vi "Read Images from File.vi"() -> ()   [LabVIEW 2023]
doc: "The Read Images from File example shows how to read images from various file types. These include a folder of image formats such as PNG, JPG, BMP, and TIFF, as well as AVI and TDMS. Use the Comparison of Streaming File Formats, Stream to AVI, Stream to Image File, or Stream to TDMS examples to create these image files."
uses:
  <vilib>/vision/Avi.llb/IMAQ AVI2 Refnum.ctl
  SubVIs/TDMS Read Data.ctl
  <vilib>/vision/Image Controls.llb/IMAQ Image.ctl
  SubVIs/TDMS File Initialization (Read).vi
panel:
  in  "Stop":bool
  in  "Image Type":u16(ring) items=["Grayscale (U8)"=0, "Grayscale (I16)"=1, "Grayscale (U16)"=7, "RGB Color (U32)"=4]
  in  "Selected Image Index":u64(slide) scale=0.0..1196.0
  out "Image":T1(plugin-control)
  in  "File Path":path
  # "Overview: Demonstrates how to read images from various file formats: image files (i.e. PNG, BMP, TIFF, etc.), AVI, and TDMS.\nRequirements: Vision Acquisition Software\nInstructions:\n1. Select the File Path to the image file to read. For image files, all images of the same type in the folder will also be read.\n2. Select the Image Type of the images saved in the file for TDMS file types. Other file types don't require this.\n3. Run the VI"
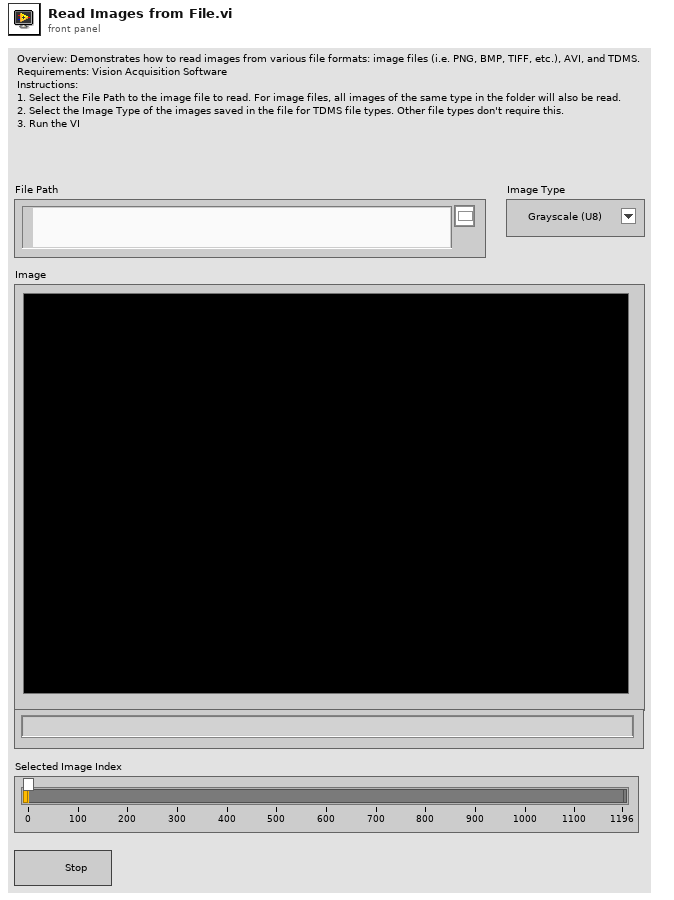
[diagram p1: front panel]
types:
  T1 = typedef "IMAQ Image.ctl" = refnum<image>
  T2 = typedef "IMAQ AVI2 Refnum.ctl" = refnum<k20>
  T3 = typedef "TDMS Read Data.ctl" = cluster{"Image Type":T4, "Width":u32, "Height":u32, "Pixels per Image":u32, "Total Width":u32, "Left Offset":u32, "Image":T1}
  T4 = typedef "Image Type" = u32
  T5 = cluster{"Image File Paths":path[], "AVI Ref":T2, "TDMS Ref":refnum<k34>, "TDMS Settings":T3}
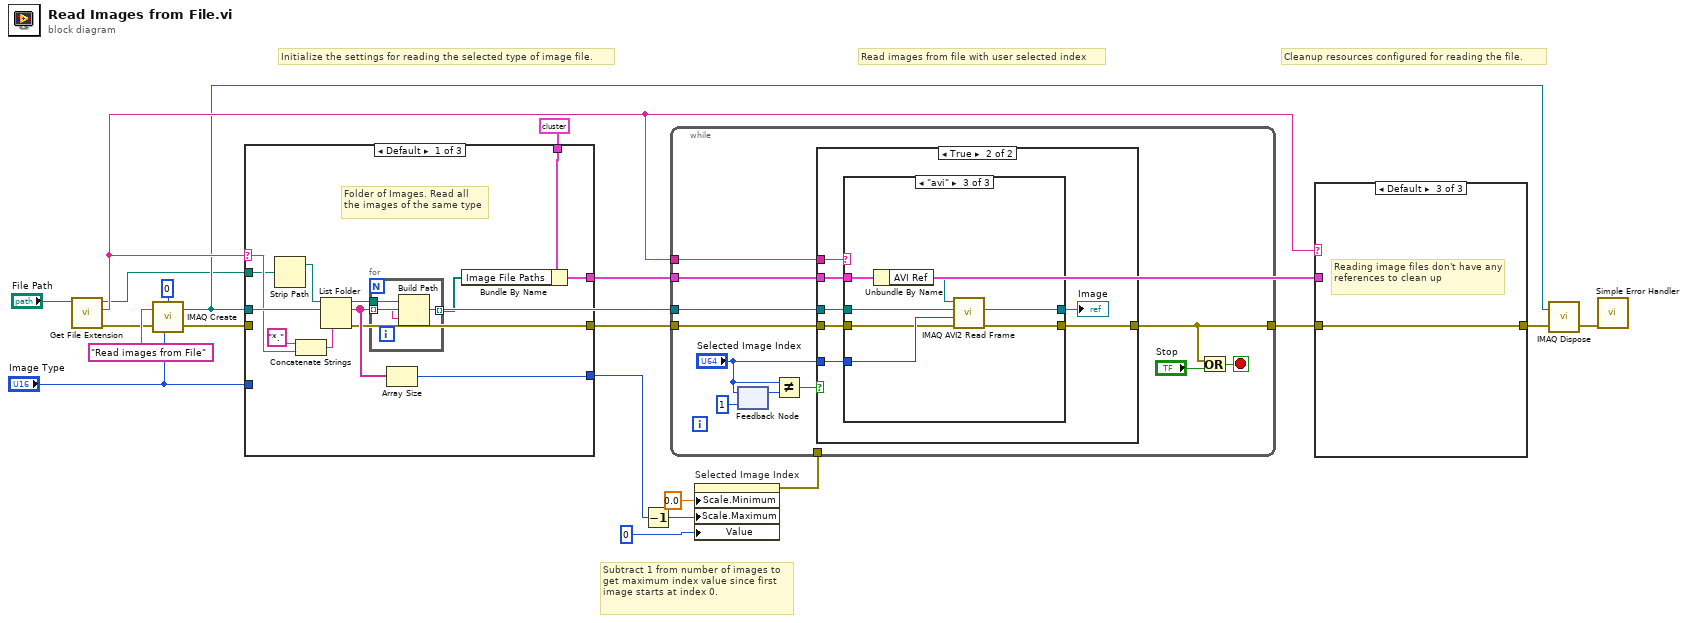
[diagram p0: block diagram]
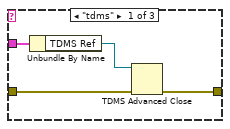
[diagram p2: hidden frame]
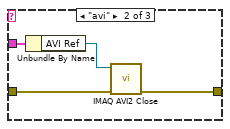
[diagram p3: hidden frame]
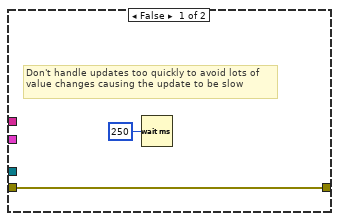
[diagram p4: hidden frame]
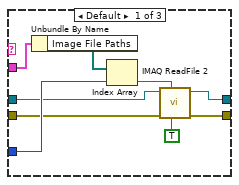
[diagram p5: hidden frame]
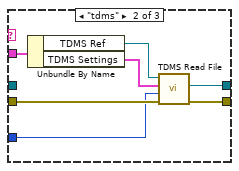
[diagram p6: hidden frame]
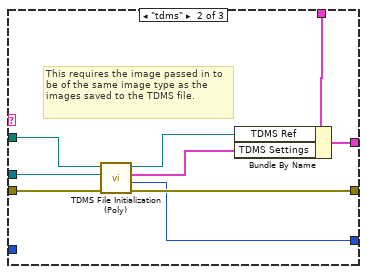
[diagram p7: hidden frame]
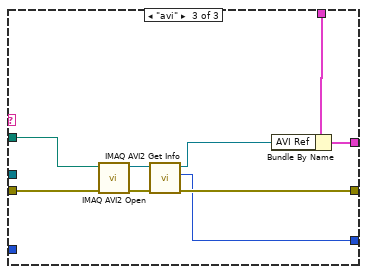
[diagram p8: hidden frame]
diagram:
  # "Subtract 1 from number of images to get maximum index value since first image starts at index 0."
  # "Cleanup resources configured for reading the file."
  # "Read images from file with user selected index"
  # "Initialize the settings for reading the selected type of image file."
  n1 = call <vilib>:"Get File Extension.vi"("file"="File Path") -> ("error out"=w2:errorcluster, "lowercase file extension"=w9:string, "dup file"=w1:path)  [unwired: 6 in, 2 out]
  n2 = call "IMAQ Create"("Border Size"=0, "Image Name"="Read images from File", "Image Type"="Image Type", "error in (no error)"=w2) -> ("New Image"=w6:T1, "error out"=w19:errorcluster)  [unwired: 1 in]
  n3 = case shown="Default" w9 {
    selector: w9 -> [w28 _ _]
    tunnel: w6 -> [_ w44 _]
    tunnel: w19 -> [_ w43 w52]
    tunnel: [w26 w42 w50] -> w15
    tunnel: w1 -> [w22 w41 w53]
    tunnel: [w30 w40 w48] -> w14
    tunnel: "Image Type" -> [_ _ _]
    tunnel: T5 {"Image File Paths"=[], "AVI Ref"=refnum, "TDMS Ref"=refnum, "TDMS Settings"={"Image Type"=0, "Width"=640, "Height"=480, "Pixels per Image"=337920, "Total Width"=640, "Left Offset"=640, "Image"="test"}} ("output cluster") -> [w25 w39 w47]
    tunnel: [w23 w36 w45] -> w8
    frame Default {
      # "Folder of Images. Read all the images of the same type"
      n4 = Strip Path(path=w22) -> (stripped path=w21:path)  [unwired: 1 out]
      n5 = Concatenate Strings("*." ("string"), w28) -> (w27:string)
      n6 = List Folder(path=w21, pattern=w27) -> (path out=w32:path, filenames=w31:string[], error out=w26:errorcluster)  [unwired: 2 in, 1 out]
      n7 = for {
        tunnel: w32 -> [w35]
        tunnel: w31 -> [w34] mode=indexing
        tunnel: [w33] -> w24 mode=indexing
        n8 = Build Path(base path=w35, name or relative path=w34) -> (appended path=w33:path)
      }
      n9 = Array Size(array=w31) -> (size(s)=w30:i32)
      n10 = Bundle By Name(cluster=w25, "Image File Paths"=w24) -> (w23:T5)
    }
    frame "tdms" {
      # "This requires the image passed in to be of the same image type as the images saved to the TDMS file."
      n11 = call-poly "TDMS File Initialization (Poly).vi"("error in (no error)"=w43, "Image In"=w44, "File Path"=w41) -> ("error out"=w42:errorcluster, "Number of Images in TDMS File"=w40:u32, "Read Settings"=w37:T3, "TDMS Refnum Out"=w38:refnum<k34>)  [unwired: 5 in]
      n12 = Bundle By Name(cluster=w39, "TDMS Ref"=w38, "TDMS Settings"=w37) -> (w36:T5)
    }
    frame "avi" {
      n13 = call "IMAQ AVI2 Open"("error in (no error)"=w52, "AVI File Path"=w53) -> ("error out"=w51:errorcluster, "AVI Refnum"=w49:T2)  [unwired: 8 in]
      n14 = call "IMAQ AVI2 Get Info"("error in (no error)"=w51, "AVI Refnum"=w49) -> ("error out"=w50:errorcluster, "Number of Frames"=w48:u32, "AVI Refnum (duplicate)"=w46:T2)  [unwired: 5 in, 2 out]
      n15 = Bundle By Name(cluster=w47, "AVI Ref"=w46) -> (w45:T5)
    }
  }
  n16 = Decrement(x=w14) -> (x-1=w3:u32)
  n17 = property on="Selected Image Index" class="Slide (strict)"("Scale.Minimum"=0.0 ("Scale.Range:Minimum"), "Scale.Maximum"=w3, "Value"=u64 0 ("Selected Image")) -> (error out=w13:errorcluster)  [unwired: 2 in, 1 out]
  n18 = while {
    tunnel: w15 -> [w64]
    tunnel: w6 -> [w57]
    tunnel: w13 -> [_]
    tunnel: w9 -> [w63]
    tunnel: w8 -> [w59]
    tunnel: [w54] -> w10
    stop <- w55 stop-if-true
    n19 = feedback-in #1("Selected Image Index") -> ()
    n20 = feedback #1(u64 1 ("Selected Image")) -> (w61:u64)
    n21 = Not Equal?(x="Selected Image Index", y=w61) -> (x != y?=w60:bool)
    n22 = case shown="True" w60 {
      tunnel: w64 -> [w65 w73]
      tunnel: w63 -> [_ w72]
      tunnel: w59 -> [_ w71]
      tunnel: "Selected Image Index" -> [_ w70]
      tunnel: w57 -> [_ w69]
      tunnel: [w65 w67] -> w54
      frame False {
        # "Don't handle updates too quickly to avoid lots of value changes causing the update to be slow"
        n23 = Wait (ms)(milliseconds to wait=u32 250) -> ()  [unwired: 1 out]
      }
      frame True {
        n24 = case shown="\"avi\"" w72 {
          tunnel: w73 -> [w76 w89 w93]
          tunnel: w71 -> [w82 w87 w96]
          tunnel: w70 -> [w80 w88 w94]
          tunnel: [w78 w84 w91] -> w68
          tunnel: [w77 w83 w90] -> w67
          tunnel: w69 -> [w75 _ w92]
          frame Default {
            n25 = Unbundle By Name(w82) -> ("Image File Paths"=w81:path[])
            n26 = Index Array(array=w81, index=w80) -> (element=w79:path)
            n27 = call "IMAQ ReadFile 2"("Use File Path Image Type"=TRUE, "File Path"=w79, "error in (no error)"=w76, "Image"=w75) -> ("error out"=w77:errorcluster, "Image Out"=w78:T1)  [unwired: 3 in, 3 out]
          }
          frame "tdms" {
            n28 = Unbundle By Name(w87) -> ("TDMS Ref"=w86:refnum<k34>, "TDMS Settings"=w85:T3)
            n29 = call "TDMS Read File.vi"("error in"=w89, "Image Index"=w88, "Read Settings"=w85, "TDMS Refnum In"=w86) -> ("error out"=w83:errorcluster, "Image"=w84:T1)  [unwired: 4 in, 2 out]
          }
          frame "avi" {
            n30 = Unbundle By Name(w96) -> ("AVI Ref"=w95:T2)
            n31 = call "IMAQ AVI2 Read Frame"("error in (no error)"=w93, "Frame Number"=w94, "Image"=w92, "AVI Refnum"=w95) -> ("error out"=w90:errorcluster, "Image Out"=w91:T1)  [unwired: 5 in, 1 out]
          }
        }
        "Image" <- w68
      }
    }
    n32 = Or(x=w54, y="Stop") -> (x .or. y?=w55:bool)
  }
  n33 = case shown="Default" w9 {
    tunnel: w10 -> [w99 w102 w105]
    tunnel: w8 -> [w100 w104 _]
    tunnel: [w97 w101 w105] -> w7
    frame "tdms" {
      n34 = Unbundle By Name(w100) -> ("TDMS Ref"=w98:refnum<k34>)
      n35 = TDMS Advanced Close(8:w99, 11:w98) -> (0:w97:errorcluster)  [unwired: 2 in, 1 out]
    }
    frame "avi" {
      n36 = Unbundle By Name(w104) -> ("AVI Ref"=w103:T2)
      n37 = call "IMAQ AVI2 Close"("error in (no error)"=w102, "AVI Refnum"=w103) -> ("error out"=w101:errorcluster)  [unwired: 9 in]
    }
    frame Default {
      # "Reading image files don't have any references to clean up"
    }
  }
  n38 = call "IMAQ Dispose"("Image"=w6, "error in (no error)"=w7) -> ("error out"=w5:errorcluster)  [unwired: 4 in]
  n39 = call <vilib>:"Simple Error Handler.vi"("error in (no error)"=w5) -> ()  [unwired: 4 in, 5 out]
